vi "Suppress Error Code - Array.vi"(8 "Error In":errorcluster, 9 "Error Codes":i32[](array[numeric])) -> (0 "Error Out":errorcluster, 1 "Error Supressed?":bool)   [LabVIEW 2012]
doc: "Clears the specific error passed in, but leaves any other untouched.\n\nFreeware from Moore Good Ideas, www.mooregoodideas.com. Do not remove this line."
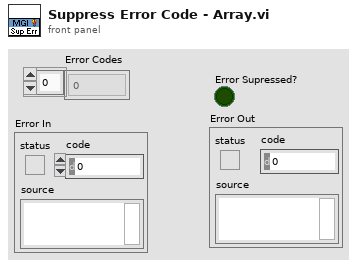
[diagram p1: front panel]
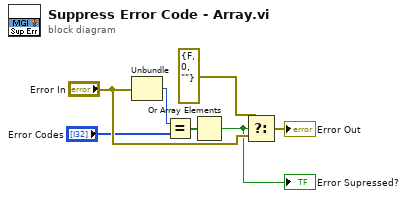
[diagram p0: block diagram]
diagram:
  n1 = Unbundle("Error In") -> ("code"=w6:i32)  [unwired: 2 out]
  n2 = Equal?(x=w6, y="Error Codes") -> (x = y?=w2:bool[])
  n3 = Or Array Elements(Boolean array=w2) -> (logical OR=w1:bool)
  "Error Supressed?" <- w1
  n4 = Select(t=errorcluster {"status"=FALSE, "code"=0, "source"=""} ("error IO"), s=w1, f="Error In") -> (s? t:f=→"Error Out":errorcluster)
